vi "Set Manual Tab Control Status.vi"(11 "Value":enum32{"Manual", "Test"}(ring)) -> ()   [LabVIEW 2020]
uses:
  support/REF Single  Name to ref convert.vi
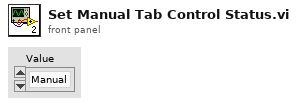
[diagram p1: front panel]
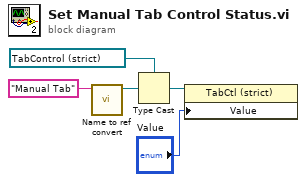
[diagram p0: block diagram]
diagram:
  n1 = call-poly "Name to ref convert.vi"("name"="Manual Tab") -> ("First REF"=w2:refnum<vi>)  [unwired: 10 in]
  n2 = Type Cast(type=refnum<vi> refnum ("Manual Tab"), x=w2) -> (*(type *) &x=w4:refnum<vi>)
  n3 = property class="TabCtl (strict)"(reference=w4, "Value"="Value") -> ()  [unwired: 1 in, 2 out]
